vi "Save FGV.vi"(8 "error in (no error)":errorcluster, 10 "Data in":dbl[](array[numeric]), 11 "CMD":enum16{"Initial", "Read", "Write", "Release"}(ring)) -> (0 "error out":errorcluster, 3 "file queue out":refnum<queue>)   [LabVIEW 2018]
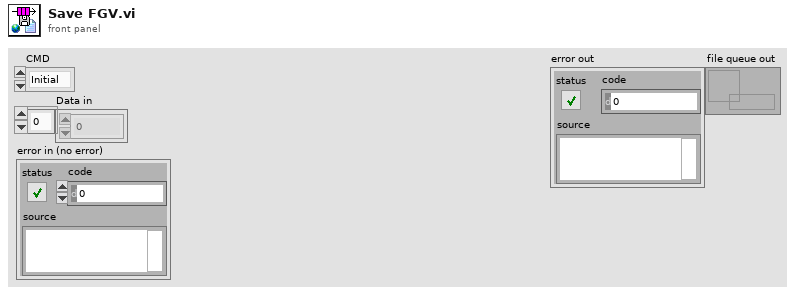
[diagram p1: front panel]
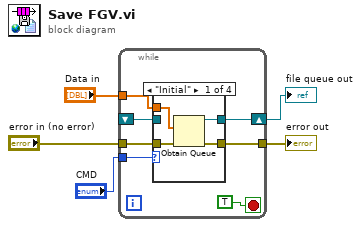
[diagram p0: block diagram]
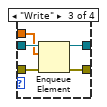
[diagram p3: hidden frame]
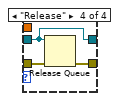
[diagram p4: hidden frame]
diagram:
  n1 = while {
    tunnel: "CMD" -> [w12]
    shift-right: [w10] -> w1
    shift-left: _ -> [w8]
    tunnel: [w9] -> w4
    tunnel: "error in (no error)" -> [w7]
    tunnel: "Data in" -> [w6]
    stop <- TRUE stop-if-true
    n2 = case shown="\"Initial\"" w12 {
      tunnel: [w16 w18 w22 w24] -> w10
      tunnel: [w14 w17 w21 w25] -> w9
      tunnel: w8 -> [_ w18 w23 w24]
      tunnel: w7 -> [w15 w17 w20 w26]
      tunnel: w6 -> [w13 _ w19 _]
      frame "Initial" {
        n3 = Obtain Queue(element data type=w13, error in (no error)=w15) -> (queue out=w16:refnum<queue>, error out=w14:errorcluster)  [unwired: 3 in, 1 out]
      }
      frame "Read" {
      }
      frame "Write" {
        n4 = Enqueue Element(queue=w23, element=w19, error in (no error)=w20) -> (queue out=w22:refnum<queue>, error out=w21:errorcluster)  [unwired: 1 in, 1 out]
      }
      frame "Release" {
        n5 = Release Queue(queue=w24, error in (no error)=w26) -> (error out=w25:errorcluster)  [unwired: 1 in, 2 out]
      }
    }
  }
  "error out" <- w4
  "file queue out" <- w1
